vi "data表转mysql日数据表.vi"(9 "YZBH":string, 10 "YZMC":string="氨氮", 11 "data":string[](array[string])) -> (3 "mysqldata簇":T1 {"JCSJ" format="%<%Y/%m/%d %H:%M:%S>T"})   [LabVIEW 2016]
panel:
  out "mysql完整簇":T2 {"JCSJ" format="%<%Y/%m/%d %H:%M:%S>T"}
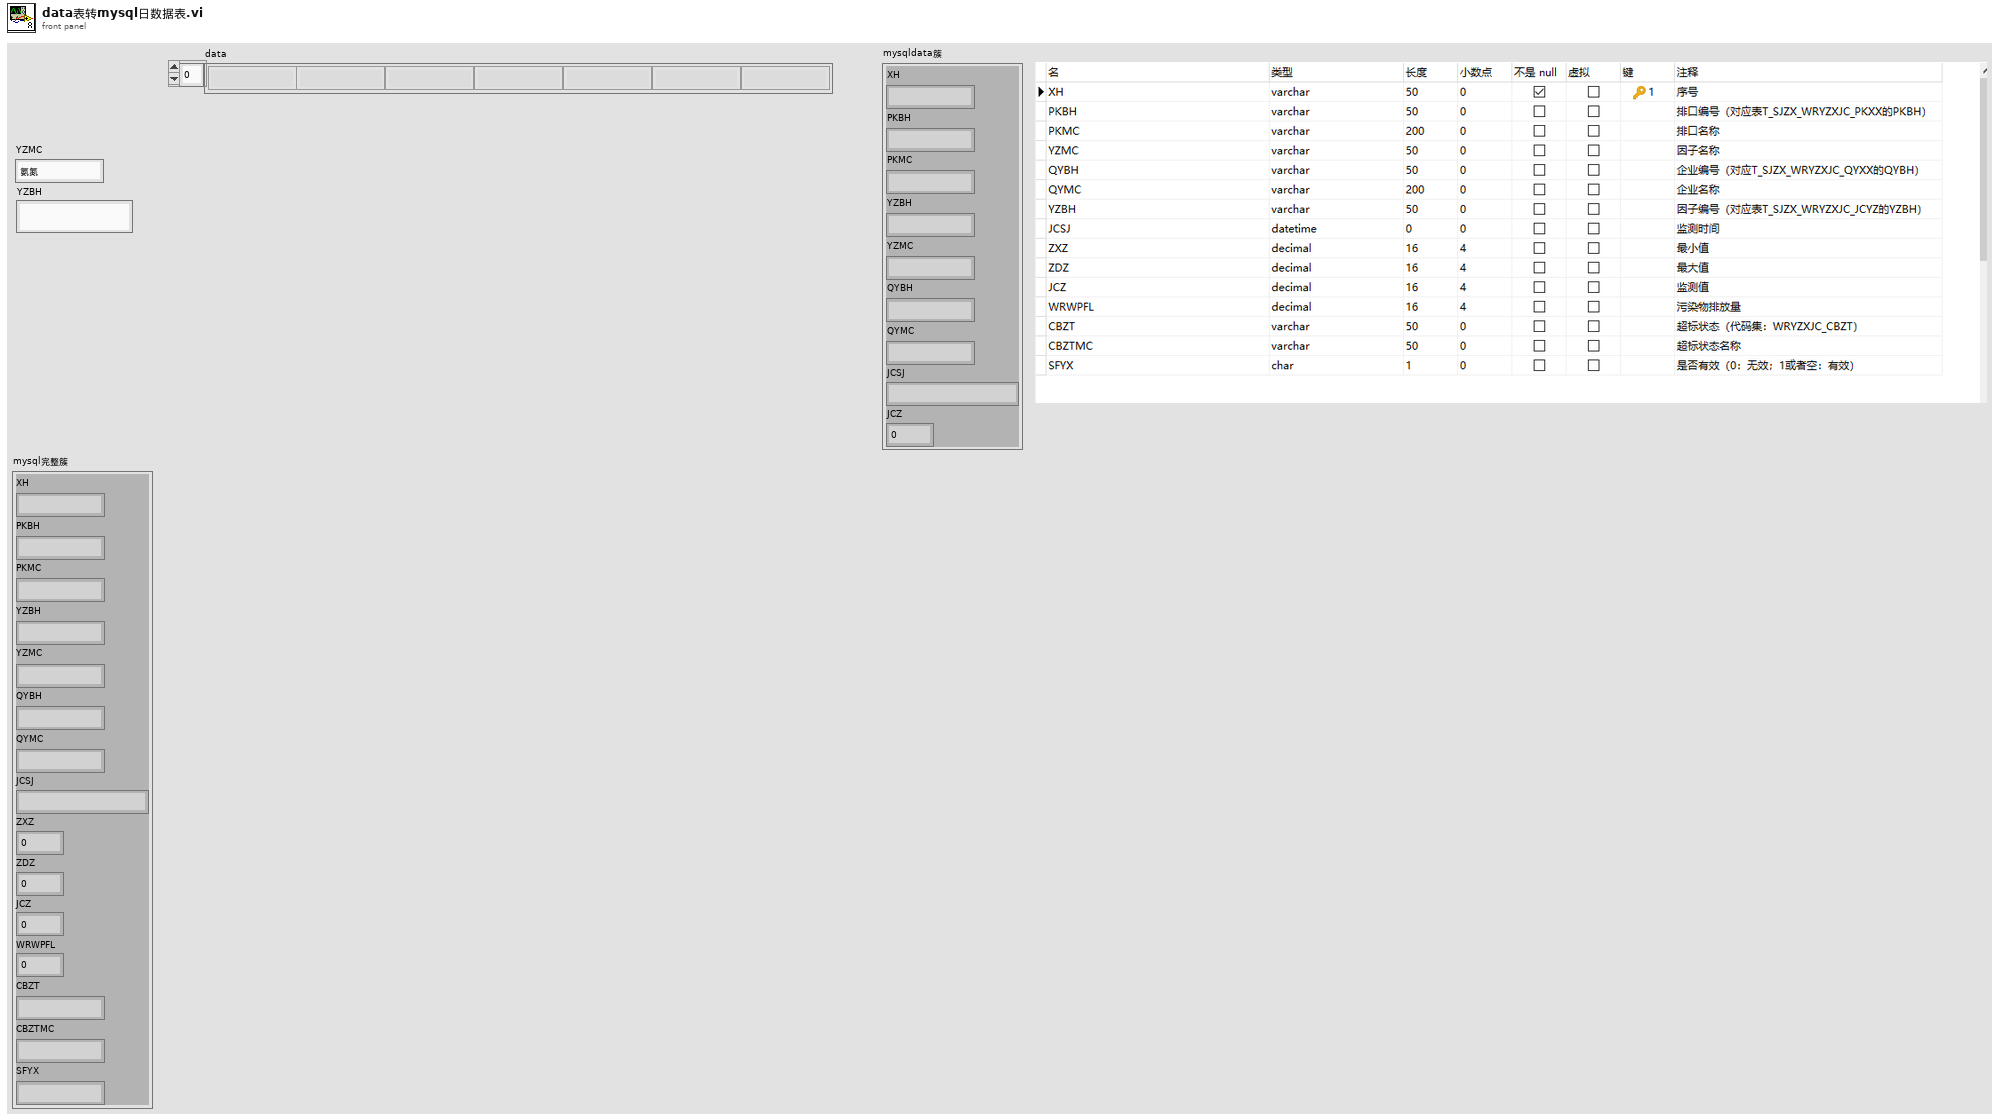
[diagram p1: front panel]
types:
  T1 = cluster{"XH":string, "PKBH":string, "PKMC":string, "YZBH":string, "YZMC":string, "QYBH":string, "QYMC":string, "JCSJ":timestamp, "JCZ":dbl}
  T2 = cluster{"XH":string, "PKBH":string, "PKMC":string, "YZBH":string, "YZMC":string, "QYBH":string, "QYMC":string, "JCSJ":timestamp, "ZXZ":dbl, "ZDZ":dbl, "JCZ":dbl, "WRWPFL":dbl, "CBZT":string, "CBZTMC":string, "SFYX":string}
  T3 = cluster{"XH":string, "PKBH":string, "PKMC":string, "YZMC":string, "QYBH":string, "QYMC":string, "YZBH":string, "JCSJ":timestamp, "JCZ":dbl}
  T4 = typedef "LVDateTimeRec.ctl" = cluster{"秒数的小数部分":dbl, "秒":i32, "分":i32, "时":i32, "日":i32, "月":i32, "年":i32, "天数（周）":i32, "天数（年）":i32, "DST":i32}
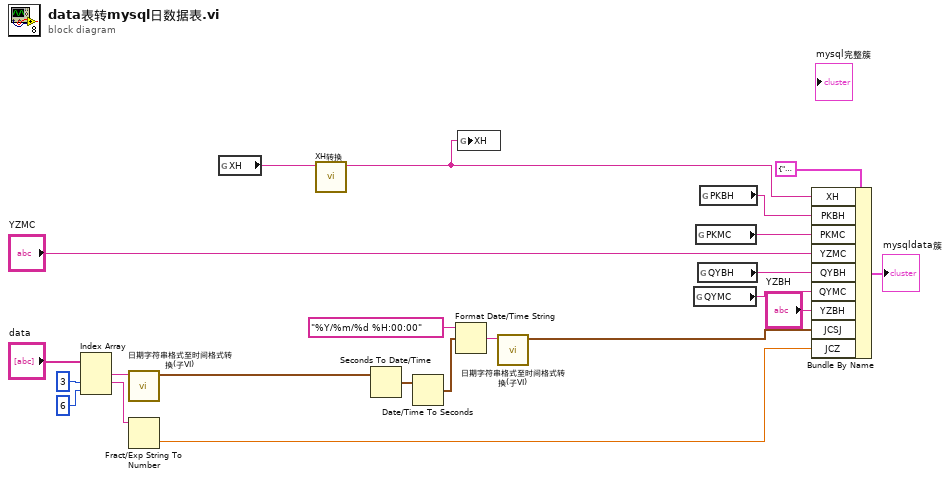
[diagram p0: block diagram]
diagram:
  n1 = Index Array(array="data", index #2=3 ("索引"), index #3=6 ("索引")) -> (element #1=w18:string, element #2=w17:string)  [unwired: 1 in, 1 out]
  n2 = call "日期字符串格式至时间格式转换(子VI).vi"("data[0]"=w18) -> ("time stamp"=w13:timestamp)  [unwired: 10 in]
  n3 = Fract/Exp String To Number(string=w17) -> (number=w16:dbl)  [unwired: 3 in, 1 out]
  n4 = global read "断电保存全局.vi" "XH"() -> (w2:string)
  n5 = call "XH转换.vi"("XH"=w2) -> ("xh输出"=w1:string)  [unwired: 10 in]
  n6 = Seconds To Date/Time(time stamp (now)=w13) -> (date time rec=w12:T4)  [unwired: 1 in]
  n7 = Date/Time To Seconds(2:w12) -> (0:w14:timestamp)  [unwired: 1 in]
  n8 = Format Date/Time String(time format string (%c)="%Y/%m/%d %H:00:00" ("时间格式字符串(%c)"), seconds (now)=w14) -> (date/time string=w11:string)  [unwired: 1 in]
  n9 = global write "断电保存全局.vi" "XH"(w1) -> ()
  n10 = call "日期字符串格式至时间格式转换(子VI).vi"("data[0]"=w11) -> ("time stamp"=w10:timestamp)  [unwired: 10 in]
  n11 = global read "断电保存全局.vi" "QYMC"() -> (w4:string)
  n12 = global read "断电保存全局.vi" "PKMC"() -> (w6:string)
  n13 = global read "断电保存全局.vi" "QYBH"() -> (w5:string)
  n14 = global read "断电保存全局.vi" "PKBH"() -> (w7:string)
  n15 = Bundle By Name(cluster=T3 {"XH"="", "PKBH"="", "PKMC"="", "YZMC"="", "QYBH"="", "QYMC"="", "YZBH"="", "JCSJ"=timestamp(0 s since 1904-01-01), "JCZ"=0.0} ("mysql簇 2"), "XH"=w1, "PKBH"=w7, "PKMC"=w6, "YZMC"="YZMC", "QYBH"=w5, "QYMC"=w4, "YZBH"="YZBH", "JCSJ"=w10, "JCZ"=w16) -> (→"mysqldata簇":T3)
